vi "Vowel-Compute Max Level.vi"(0 "Vowel In":T1, 9 "Level":T2, 11 "error in (no error)":errorcluster, 12 "Fs (Hz)":dbl) -> (4 "Vowel Out":T1, 6 "Max Level":dbl, 10 "Level out":T2, 15 "error out":errorcluster)   [LabVIEW 2020]
uses:
  XControls/Waveform XControls/Vowel/Vowel.Properties.ctl
  XControls/Level (G3)/Level Data.ctl
  XControls/Level (G3)/Level Units (G3).ctl
  Utility VIs/Math VIs/Linear to dB (scalar).vi
  PXI DAQ VIs/DAQ Engine VIs/PXI Globals.vi
  Utility VIs/Math VIs/interp1 (1D).vi
  Utility VIs/Math VIs/dB to Linear (1D).vi
  XControls/Level (G3)/Level (G3).xctl
  XControls/Waveform XControls/Vowel/Vowel.xctl
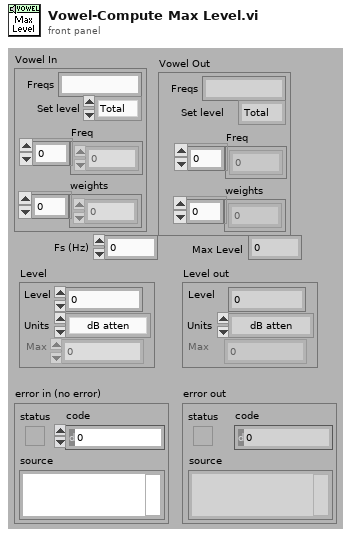
[diagram p1: front panel]
types:
  T1 = typedef "Vowel.xctl/Vowel.Properties.ctl" = cluster{"Freqs":string, "Set level":enum16{"Total", "Per component"}, "Freq":dbl[], "weights":dbl[]}
  T2 = typedef "Level (G3).xctl/Level Data.ctl" = cluster{"Level":dbl, "Units":T3, "Max":dbl, "Data":cluster{"Multiplier":dbl, "Cal File":path, "Cal":cluster{"Freq (Hz)":dbl[], "Mag (dB SPL)":dbl[], "Phase (deg)":dbl[]}, "audiogram":path}}
  T3 = typedef "Level (G3).xctl/Level Units (G3).ctl" = enum16{"dB atten", "dB SPL", "dB re 1 Vrms", "dB V/Hz½", "mW", "dB HL", "Volts", "dB mW"}
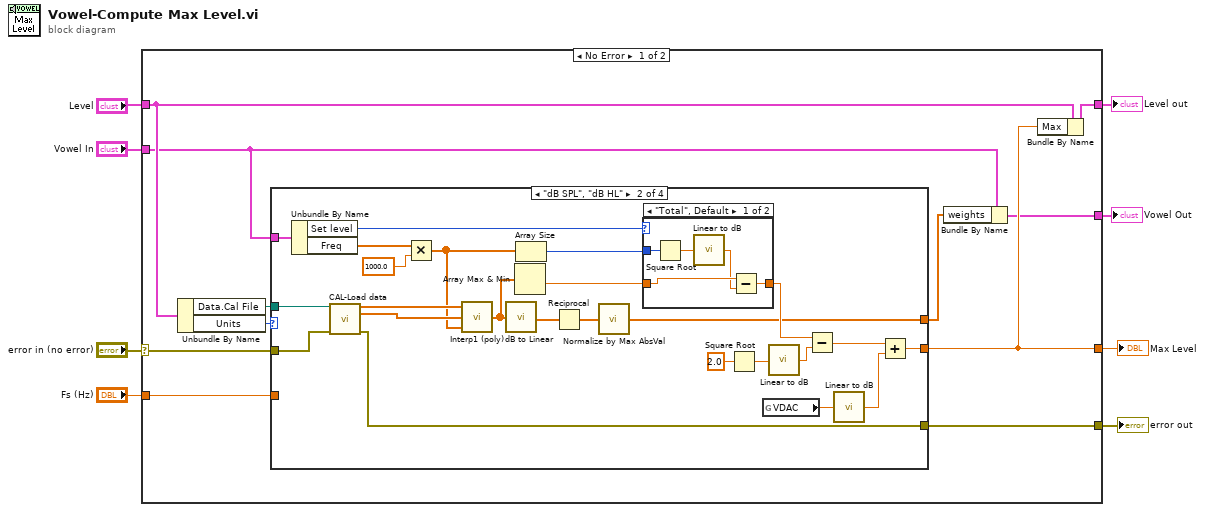
[diagram p0: block diagram]
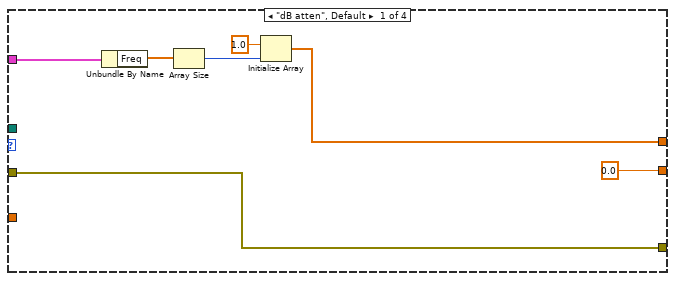
[diagram p2: hidden frame]
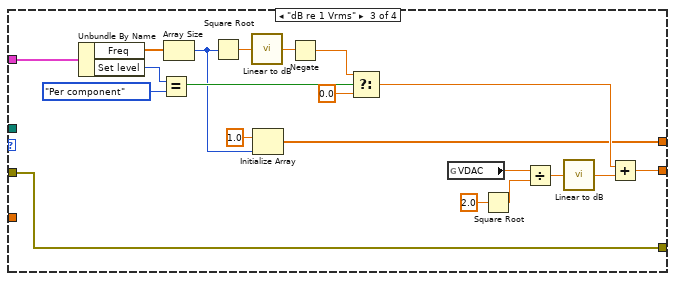
[diagram p4: hidden frame]
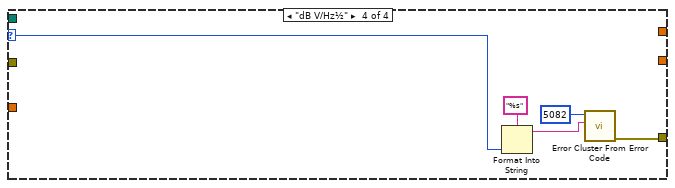
[diagram p5: hidden frame]
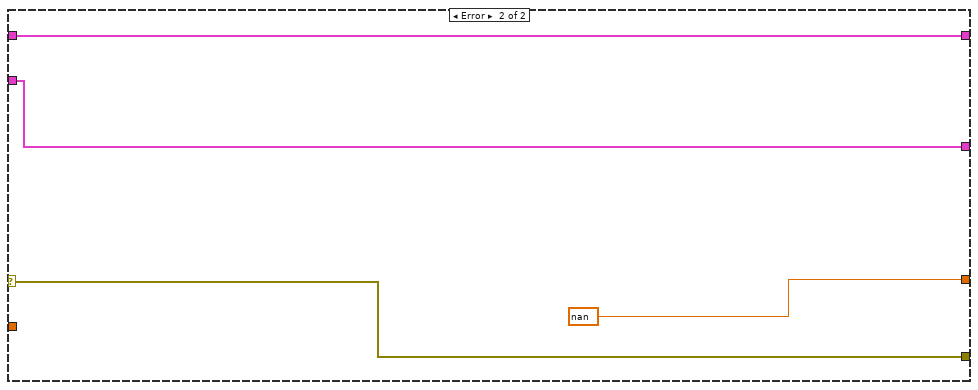
[diagram p6: hidden frame]
diagram:
  n1 = case shown="No Error" "error in (no error)" {
    selector: "error in (no error)" -> [w19 w85]
    tunnel: "Level" -> [w17 w83]
    tunnel: "Vowel In" -> [w11 w82]
    tunnel: [w18 w85] -> w7
    tunnel: [w16 nan ("Reference Level")] -> w4
    tunnel: [w15 w83] -> w3
    tunnel: "Fs (Hz)" -> [w12 _]
    tunnel: [w10 w82] -> w1
    frame No Error {
      n2 = Unbundle By Name(w17) -> ("Data.Cal File"=w14:path, "Units"=w13:T3)
      n3 = case shown="\"dB SPL\", \"dB HL\"" w13 {
        selector: w13 -> [_ _ _ w77]
        tunnel: w19 -> [w25 w50 w76 _]
        tunnel: w11 -> [w21 w48 w70 _]
        tunnel: [0.0 ("Reference Level") w49 w67 _] -> w16
        tunnel: [w25 w47 w76 w78] -> w18
        tunnel: w14 -> [_ w46 _ _]
        tunnel: w12 -> [_ _ _ _]
        tunnel: [w20 w27 w57 _] -> w9
        frame "dB atten", Default {
          n4 = Unbundle By Name(w21) -> ("Freq"=w24:dbl[])
          n5 = Array Size(array=w24) -> (size(s)=w23:i32)
          n6 = Initialize Array(1.0 ("element"), w23) -> (w20:dbl[])
        }
        frame "dB SPL", "dB HL" {
          n7 = Unbundle By Name(w48) -> ("Set level"=w32:enum16{"Total", "Per component"}, "Freq"=w43:dbl[])
          n8 = call "CAL-Load data.vi"("user path"=w46, "error in (no error)"=w50) -> ("Frequency (Hz)"=w37:dbl[], "Mag"=w36:dbl[], "error out"=w47:errorcluster)  [unwired: 6 in, 5 out]
          n9 = Multiply(x=w43, y=1000.0) -> (x*y=w29:dbl[])
          n10 = call-poly "Interp1 (poly).vi"("X"=w37, "Y"=w36, "U"=w29) -> ("V"=w33:dbl[])  [unwired: 2 in]
          n11 = call-poly "dB to Linear.vi"("dB"=w33) -> ("linear"=w35:dbl[])
          n12 = Array Max & Min(array=w33) -> (min value=w31:dbl)  [unwired: 3 out]
          n13 = Array Size(array=w29) -> (size(s)=w28:i32)
          n14 = Reciprocal(x=w35) -> (1/x=w34:dbl[])
          n15 = call "Normalize by Max AbsVal.vi"("Y"=w34) -> ("Ynorm"=w27:dbl[])
          n16 = case shown="\"Total\", Default" w32 {
            tunnel: w31 -> [w52 w56]
            tunnel: [w53 w56] -> w30
            tunnel: w28 -> [w55 _]
            frame "Total", Default {
              n17 = Square Root(x=w55) -> (sqrt(x)=w54:dbl)
              n18 = call-poly "Linear to dB.vi"("Linear"=w54) -> ("dB"=w51:dbl)
              n19 = Subtract(x=w52, y=w51) -> (x-y=w53:dbl)
            }
            frame "Per component" {
            }
          }
          n20 = Square Root(x=2.0 ("y")) -> (sqrt(x)=w40:dbl)
          n21 = global read "PXI Globals.vi" "VDAC"() -> (w45:dbl)
          n22 = call-poly "Linear to dB.vi"("Linear"=w40) -> ("dB"=w39:dbl)
          n23 = Subtract(x=w30, y=w39) -> (x-y=w38:dbl)
          n24 = call-poly "Linear to dB.vi"("Linear"=w45) -> ("dB"=w44:dbl)
          n25 = Add(x=w38, y=w44) -> (x+y=w49:dbl)
        }
        frame "dB re 1 Vrms" {
          n26 = Unbundle By Name(w70) -> ("Freq"=w69:dbl[], "Set level"=w66:enum16{"Total", "Per component"})
          n27 = Equal?(x=w66, y=enum16{"Total", "Per component"}."Per component") -> (x = y?=w64:bool)
          n28 = Array Size(array=w69) -> (size(s)=w59:i32)
          n29 = Square Root(x=w59) -> (sqrt(x)=w68:dbl)
          n30 = call-poly "Linear to dB.vi"("Linear"=w68) -> ("dB"=w61:dbl)
          n31 = Initialize Array(1.0 ("element"), w59) -> (w57:dbl[])
          n32 = Negate(x=w61) -> (-x=w60:dbl)
          n33 = Select(t=w60, s=w64, f=0.0) -> (s? t:f=w62:dbl)
          n34 = global read "PXI Globals.vi" "VDAC"() -> (w73:dbl)
          n35 = Square Root(x=2.0 ("y")) -> (sqrt(x)=w74:dbl)
          n36 = Divide(x=w73, y=w74) -> (x/y=w72:dbl)
          n37 = call-poly "Linear to dB.vi"("Linear"=w72) -> ("dB"=w71:dbl)
          n38 = Add(x=w62, y=w71) -> (x+y=w67:dbl)
        }
        frame "dB V/Hz½" {
          n39 = Format Into String(format string="%s", w77) -> (resulting string=w80:string)  [unwired: 2 in, 1 out]
          n40 = call <vilib>:"Error Cluster From Error Code.vi"("error message (\"\")"=w80, "error code (0)"=5082) -> ("error out"=w78:errorcluster)  [unwired: 7 in]
        }
      }
      n41 = Bundle By Name(cluster=w11, "weights"=w9) -> (w10:T1)
      n42 = Bundle By Name(cluster=w17, "Max"=w16) -> (w15:T2)
    }
    frame Error {
    }
  }
  "error out" <- w7
  "Max Level" <- w4
  "Level out" <- w3
  "Vowel Out" <- w1
